vi "Write Timeout Message.vi"(8 "Timeout Message Priority (Normal)":T1=enum."Normal", 9 "Timeout [ms]":i32=-1, 10 "Timeout Message":refnum<class "Message.lvclass">, 11 "IEventHandler in":refnum<class "IEventHandler.lvclass">) -> (3 "IEventHandler out":refnum<class "IEventHandler.lvclass">)   [LabVIEW 2015, in "ActorEvents.lvlib" / "IEventHandler.lvclass"]
uses:
  IEventHandler.lvclass
  <vilib>/ActorFramework/Message/Message.lvclass
  <vilib>/ActorFramework/Message Enqueuer/Message Priority.ctl
  IEventHandler.lvclass/IEventHandler.ctl
  <vilib>/ActorFramework/Message Enqueuer/Message Enqueuer.lvclass
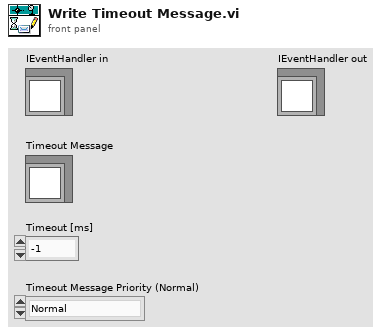
[diagram p1: front panel]
types:
  T1 = typedef "Actor Framework.lvlib/Message Enqueuer.lvclass/Message Priority.ctl" = enum16{"Low", "Normal", "High"}
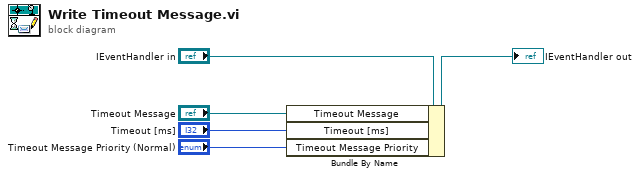
[diagram p0: block diagram]
diagram:
  n1 = Bundle By Name(cluster="IEventHandler in", "Timeout Message"="Timeout Message", "Timeout [ms]"="Timeout [ms]", "Timeout Message Priority"="Timeout Message Priority (Normal)") -> (→"IEventHandler out":refnum<class "IEventHandler.lvclass">)
